vi "nominal run update commit.vi"(7 "out_run":i32, 8 "error in (no error)":errorcluster, 9 "staging":i32, 10 "rid":string, 11 "client":i32) -> (0 "error out":errorcluster, 3 "function return":i32, 5 "out_run out":i32)   [LabVIEW 2020, in "client.lvlib"]
doc: "int32_t nominal_run_update_commit(int32_t client,\n const char *rid,\n int32_t staging,\n int32_t *out_run);"
uses:
  client.lvlib
  nominalClient_64.dll
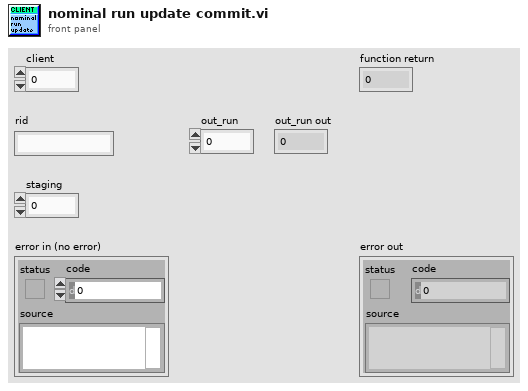
[diagram p1: front panel]
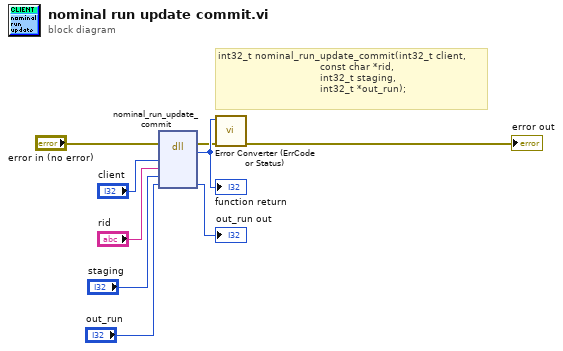
[diagram p0: block diagram]
diagram:
  # "int32_t nominal_run_update_commit(int32_t client,\n                                  const char *rid,\n                                  int32_t staging,\n                                  int32_t *out_run);"
  n1 = dll-call lib="C:/code/labview-client-rs/lv_src/client/nominalClient_*.dll" fn="nominal_run_update_commit"(error in="error in (no error)", "client"="client", "rid"="rid", "staging"="staging", "out_run"="out_run") -> (error out=w2:errorcluster, w9:i32, "out_run"=→"out_run out":i32)  [unwired: 5 in, 1 out]
  "function return" <- w9
  n2 = call "Error Converter (ErrCode or Status).vi"("error in (no error)"=w2, "error code"=w9) -> ("error out"=→"error out":errorcluster)  [unwired: 9 in]
